vi "Display Timeout Two Button Popup.vi"(5 "N-Text":string="No", 6 "Theme":refnum<class "Theme.lvclass">, 7 "Y-Text":string="Yes", 8 "error in":errorcluster, 9 "Timeout (s)":dbl=1.0 min=1.0, 10 "Message":string, 11 "Graphic":T1="info") -> (0 "error out":errorcluster, 1 "Choice":bool, 2 "Timeout":bool)   [LabVIEW 2021, in "Pop-Up.lvlib" / "Timeout Two Button.lvclass"]
doc: "The two button popup will display information to the user and wait for the operator to click the button or until time expires.\n\n<b>Note:</b> if the user does not make a selection before the timeout, the choice will output False\n\n<b>Note:</b> The function <b>Close Pop-Up (Two Button Choice).vi</b> can be used to close this dialog early and send a value for the choice. Otherwise, use Close Pop-Up.vi to close this dialog early.\n\nInputs:\n-Graphic [typedef combobox] - Image (PNG) for Graphic for Popup\n-Message [String] - String Variable to populate Display\n-Theme [lvclass] - the theme for the style of the popup\n-Y-Text [string] - the string for the YES button\n-N-Text [string] - the string for the NO button\n-Timeout (s) [DBL] - the timeout duration\n\nOutputs\n-Choice? [Boolean] - the user's button selection (YText = True, NText = False)\n\n<b>Code Developed By:</b>\nDaniel Coons\nTechnology Service Corporation\n1983 S Liberty Drive\nBloomington, IN 47403\nPhone: 812 558-7100\ndaniel.coons@tsc.com\nwww.tsc.com/atcs"
uses:
  Timeout Two Button.lvclass
  Theme/Theme.lvclass
  Graphics.ctl
  C:/Development/Open Source/tsc-pop-up/Popup/Popup.lvclass
  Timeout Two Button.lvclass/Timeout Two Button.ctl
  Popup/Popup.lvclass/Popup.ctl
  Popup/Popup.lvclass
  Pop-Up.lvlib
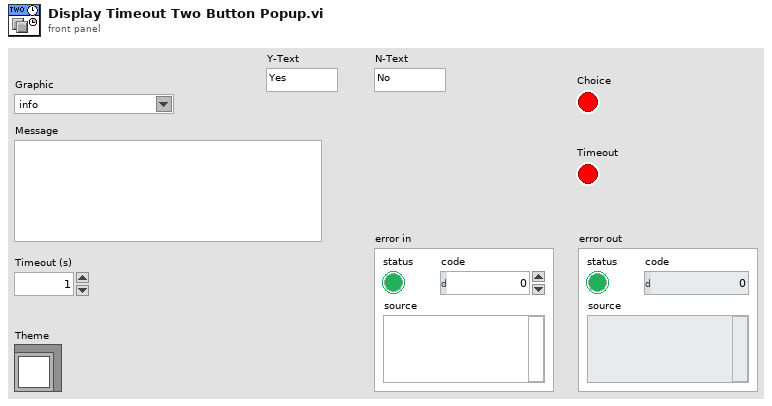
[diagram p1: front panel]
types:
  T1 = typedef "Pop-Up.lvlib/Graphics.ctl" = string
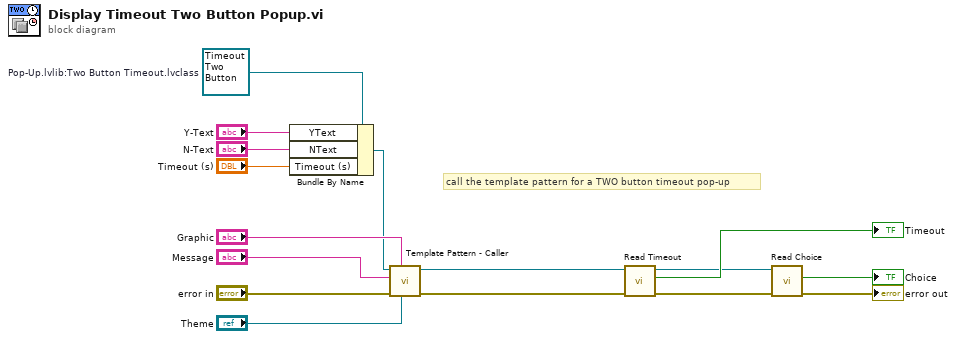
[diagram p0: block diagram]
diagram:
  w7 = refnum<class "Timeout Two Button.lvclass"> refnum  # Pop-Up.lvlib:Two Button Timeout.lvclass
  # "call the template pattern for a TWO button timeout pop-up"
  n1 = Bundle By Name(cluster=w7, "YText"="Y-Text", "NText"="N-Text", "Timeout (s)"="Timeout (s)") -> (w6:refnum<class "Timeout Two Button.lvclass">)
  n2 = call-dynamic "Template Pattern - Caller.vi"("Theme"="Theme", "standard"="Graphic", "error in (no error)"="error in", "Message"="Message", "Pop-Up in"=w6) -> ("error out"=w5:errorcluster, "Pop-Up out"=w3:refnum<class "Timeout Two Button.lvclass">)  [unwired: 5 in]
  n3 = call "Read Timeout.vi"("error in (no error)"=w5, "Popup in"=w3) -> ("error out"=w4:errorcluster, "Timeout?"=→"Timeout":bool, "Popup out"=w1:refnum<class "Timeout Two Button.lvclass">)  [unwired: 7 in]
  n4 = call-dynamic "Read Choice.vi"("error in (no error)"=w4, "_Popup in"=w1) -> ("error out"=→"error out":errorcluster, "Choice"=→"Choice":bool)  [unwired: 7 in, 1 out]
